vi "Write Pulse Configuration.vi"(8 "error in (no error)":errorcluster, 10 "Configuration":T1={"Post-trigger delay"=0.01, "Post-trigger duration"=0.1, "Rate"=1000000.0, "Ranges"=[10.0], "Re-name channels"=[], "Active channels"="0:1", "External clock"=FALSE} {"Rate" format="%#_8pHz"; "Post-trigger duration" format="%#_6ps"; "Post-trigger delay" format="%#_6ps"; "Ranges" format="%#_6pV"}, 11 "DAQmx Lockin Digitizer Driver in":refnum<class "Lockin Digitizer Driver.lvclass">) -> (0 "error out":errorcluster, 3 "DAQmx Lockin Digitizer Driver in":refnum<class "Lockin Digitizer Driver.lvclass">)   [LabVIEW 2021, in "Lockin Digitizer Driver.lvclass"]
uses:
  Lockin Digitizer Driver.lvclass
  Pusle Driver Configuration.ctl
  Lockin Digitizer Driver.lvclass/Lockin Digitizer Driver.ctl
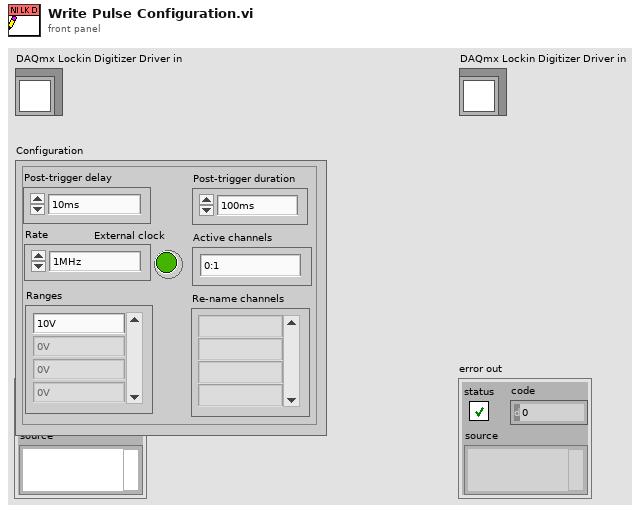
[diagram p1: front panel]
types:
  T1 = typedef "Pusle Driver Configuration.ctl" = cluster{"Post-trigger delay":dbl, "Post-trigger duration":dbl, "Rate":dbl, "Ranges":dbl[], "Re-name channels":string[], "Active channels":string, "External clock":bool}
  T2 = typedef "Lockin Digitizer Configuration.ctl" = cluster{"Post-trigger delay":dbl, "Post-trigger duration":dbl, "Rate":dbl, "Ranges":dbl[], "Re-name channels":string[], "Active channels":string, "External\nclock":bool, "Frequencies":dbl[], "Monitor time\nconstant":dbl, "Output \namplitudes":dbl[], "Input\nchannles":string[], "Sync":bool, "Lock-in input channel phases":dbl[]}
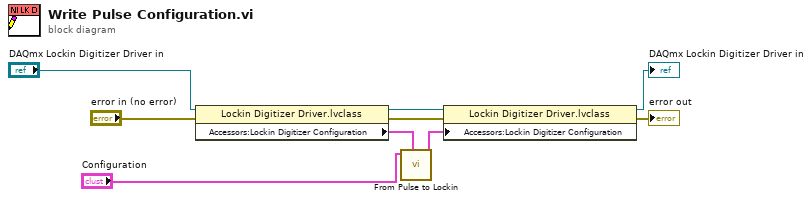
[diagram p0: block diagram]
diagram:
  n1 = property class="Lockin Digitizer Driver.lvclass"(reference="DAQmx Lockin Digitizer Driver in", error in="error in (no error)") -> (reference out=w6:refnum<class "Lockin Digitizer Driver.lvclass">, error out=w7:errorcluster, "Accessors:Lockin Digitizer Configuration"=w2:T2)
  n2 = call "From Pulse to Lockin.vi"("Lockin Configuration in"=w2, "Pulse Configuration in"="Configuration") -> ("Lockin Configuration out"=w1:T2)  [unwired: 9 in]
  n3 = property class="Lockin Digitizer Driver.lvclass"(reference=w6, error in=w7, "Accessors:Lockin Digitizer Configuration"=w1) -> (reference out=→"DAQmx Lockin Digitizer Driver in":refnum<class "Lockin Digitizer Driver.lvclass">, error out=→"error out":errorcluster)
